vi "Ventilator.vi"(0 "task_num":i32=50) -> ()   [LabVIEW 2014]
uses:
  <vilib>/addons/zeromq/socket_type.ctl
  <vilib>/addons/zeromq/zmq_context.lvclass
  <vilib>/addons/zeromq/zeromq.lvlib
  <vilib>/addons/zeromq/zmq_socket.lvclass
panel:
  in  "start":bool
  out "Estimated time: %d ms":u32
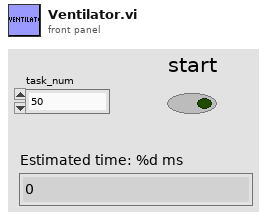
[diagram p1: front panel]
types:
  T1 = typedef "zeromq.lvlib/socket_type.ctl" = enum8{"ZMQ_PAIR", "ZMQ_PUB", "ZMQ_SUB", "ZMQ_REQ", "ZMQ_REP", "ZMQ_DEALER", "ZMQ_ROUTER", "ZMQ_PULL", "ZMQ_PUSH", "ZMQ_XPUB", "ZMQ_XSUB"}
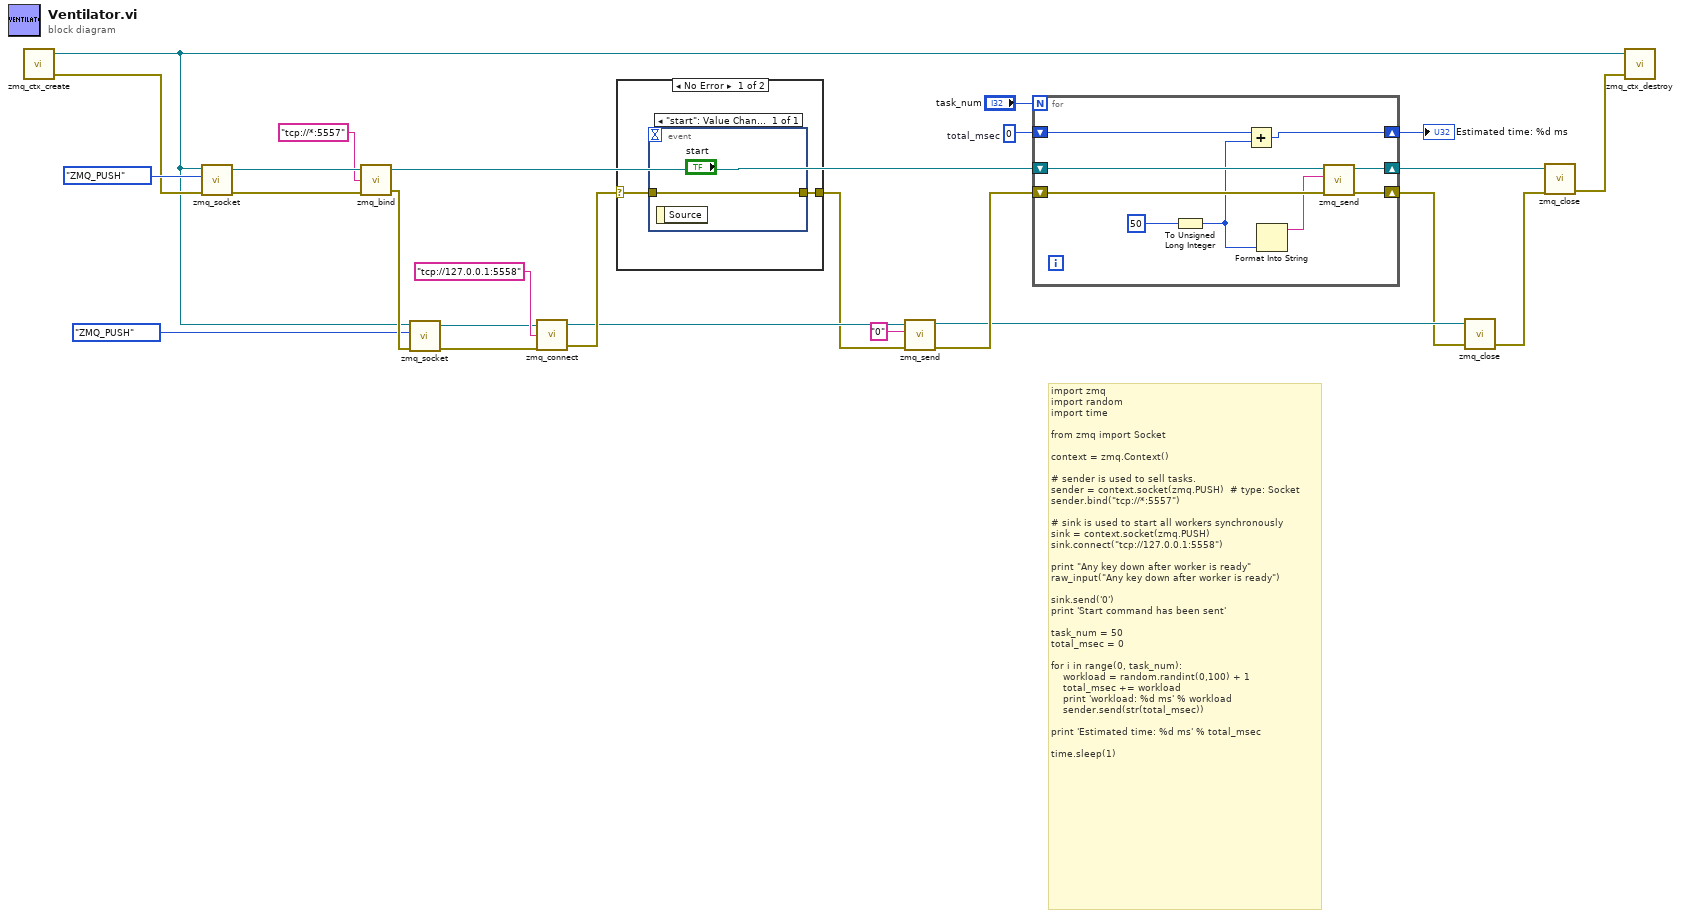
[diagram p0: block diagram]
diagram:
  w7 = 0  # total_msec
  # "import zmq\nimport random\nimport time\n\nfrom zmq import Socket\n\ncontext = zmq.Context()\n\n# sender is used to sell tasks.\nsender = context.socket(zmq.PUSH)  # type: Socket\nsender.bind(\"tcp://*:5557\")\n\n# sink is used to start all workers synchronously\nsink = context.socket(zmq.PUSH)\nsink.connect(\"tcp://127.0.0.1:5558\")\n\nprint \"Any key down after worker is ready\"\nraw_input(\"Any key down after worker is ready\")\n\nsink.send('0')\nprint 'Start command has been sent'\n\ntask_num = 50\ntotal_msec = 0\n\nfor i in range(0, task_num):\n    workload = random.randint(0,100) + 1\n    total_msec += workload\n    print 'workload: %d ms' % workload\n    sender.send(str(total_msec))\n\nprint 'Estimated time: %d ms' % total_msec\n\ntime.sleep(1)"
  n1 = call <vilib>:"zmq_ctx_create.vi"() -> ("error out"=w15:errorcluster, "context out"=w2:refnum<class "zmq_context.lvclass">)  [unwired: 4 in]
  n2 = call <vilib>:"zmq_socket.vi"("error in"=w15, "socket type"=socket_type."ZMQ_PUSH", "context in"=w2) -> ("error out"=w23:errorcluster, "socket out"=w24:refnum<class "zmq_socket.lvclass">)  [unwired: 2 in, 1 out]
  n3 = call <vilib>:"zmq_bind.vi"("error in"=w23, "endpoint"="tcp://*:5557", "socket in"=w24) -> ("error out"=w10:errorcluster, "socket out"=w21:refnum<class "zmq_socket.lvclass">)  [unwired: 1 in]
  n4 = call <vilib>:"zmq_socket.vi"("error in"=w10, "socket type"=socket_type."ZMQ_PUSH", "context in"=w2) -> ("error out"=w17:errorcluster, "socket out"=w16:refnum<class "zmq_socket.lvclass">)  [unwired: 2 in, 1 out]
  n5 = call <vilib>:"zmq_connect.vi"("error in"=w17, "endpoint"="tcp://127.0.0.1:5558", "socket in"=w16) -> ("error out"=w14:errorcluster, "socket out"=w13:refnum<class "zmq_socket.lvclass">)  [unwired: 1 in]
  n6 = case shown="No Error" w14 {
    selector: w14 -> [w27 w29]
    tunnel: [w26 w29] -> w11
    frame No Error {
      n7 = event shown="[0] \"start\": Value Change" {
        selector: _ -> [_]
        dyn-events: _ -> [_]
        timeout: _ -> [_]
        tunnel: [w28] -> w26
        tunnel: w27 -> [w28]
        event "start": Value Change {
          n8 = event-data() -> ()  [unwired: 1 in, 1 out]
        }
      }
    }
    frame Error {
    }
  }
  n9 = call <vilib>:"zmq_send.vi"("error in"=w11, "data"="0", "socket in"=w13) -> ("error out"=w8:errorcluster, "socket out"=w5:refnum<class "zmq_socket.lvclass">)  [unwired: 4 in]
  n10 = for {
    N: "task_num" -> [_]
    shift-right: [w37] -> w20
    shift-left: w21 -> [w38]
    shift-right: [w36] -> w4
    shift-left: w8 -> [w35]
    shift-right: [w33] -> w6
    shift-left: w7 -> [w34]
    n11 = To Unsigned Long Integer(number=u32 50) -> (unsigned 32bit integer=w32:u32)
    n12 = Add(x=w34, y=w32) -> (x+y=w33:u32)
    n13 = Format Into String(w32) -> (resulting string=w31:string)  [unwired: 3 in, 1 out]
    n14 = call <vilib>:"zmq_send.vi"("error in"=w35, "data"=w31, "socket in"=w38) -> ("error out"=w36:errorcluster, "socket out"=w37:refnum<class "zmq_socket.lvclass">)  [unwired: 4 in]
  }
  "Estimated time: %d ms" <- w6
  n15 = call <vilib>:"zmq_close.vi"("error in"=w4, "socket"=w5) -> ("error out"=w3:errorcluster)  [unwired: 3 in]
  n16 = call <vilib>:"zmq_close.vi"("error in"=w3, "socket"=w20) -> ("error out"=w19:errorcluster)  [unwired: 3 in]
  n17 = call <vilib>:"zmq_ctx_destroy.vi"("error in"=w19, "context in"=w2) -> ()  [unwired: 3 in, 1 out]
